vi "Newmark-GotoAll.vi"(0 "Table VRN IN":refnum<visa-resource-name>="COM9", 1 "BrasPesto":bool, 2 "Bool Refnum":refnum<vi>, 3 "LimXPesto":dbl, 7 "Notify?":bool, 11 "Error IN":errorcluster, 12 "Position X":dbl, 13 "Position Y":dbl, 14 "Position Z":dbl) -> (4 "Table VRN OUT":refnum<visa-resource-name>="COM9", 15 "Error OUT":errorcluster)   [LabVIEW 2019]
uses:
  Comm/SerialCommError.vi
panel:
  out "LimXPesto 2":dbl=54.5268 caption="Limit X avec Pesto" format="%.2f"
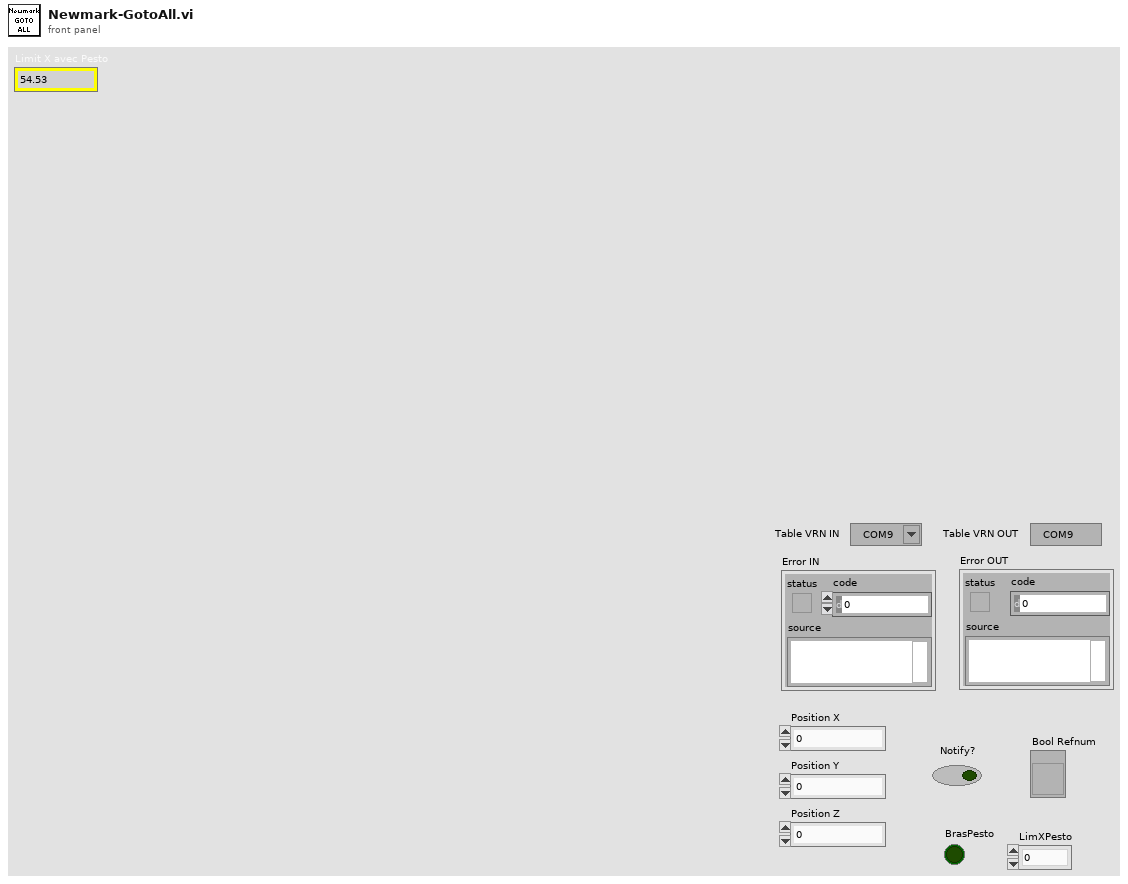
[diagram p1: front panel]
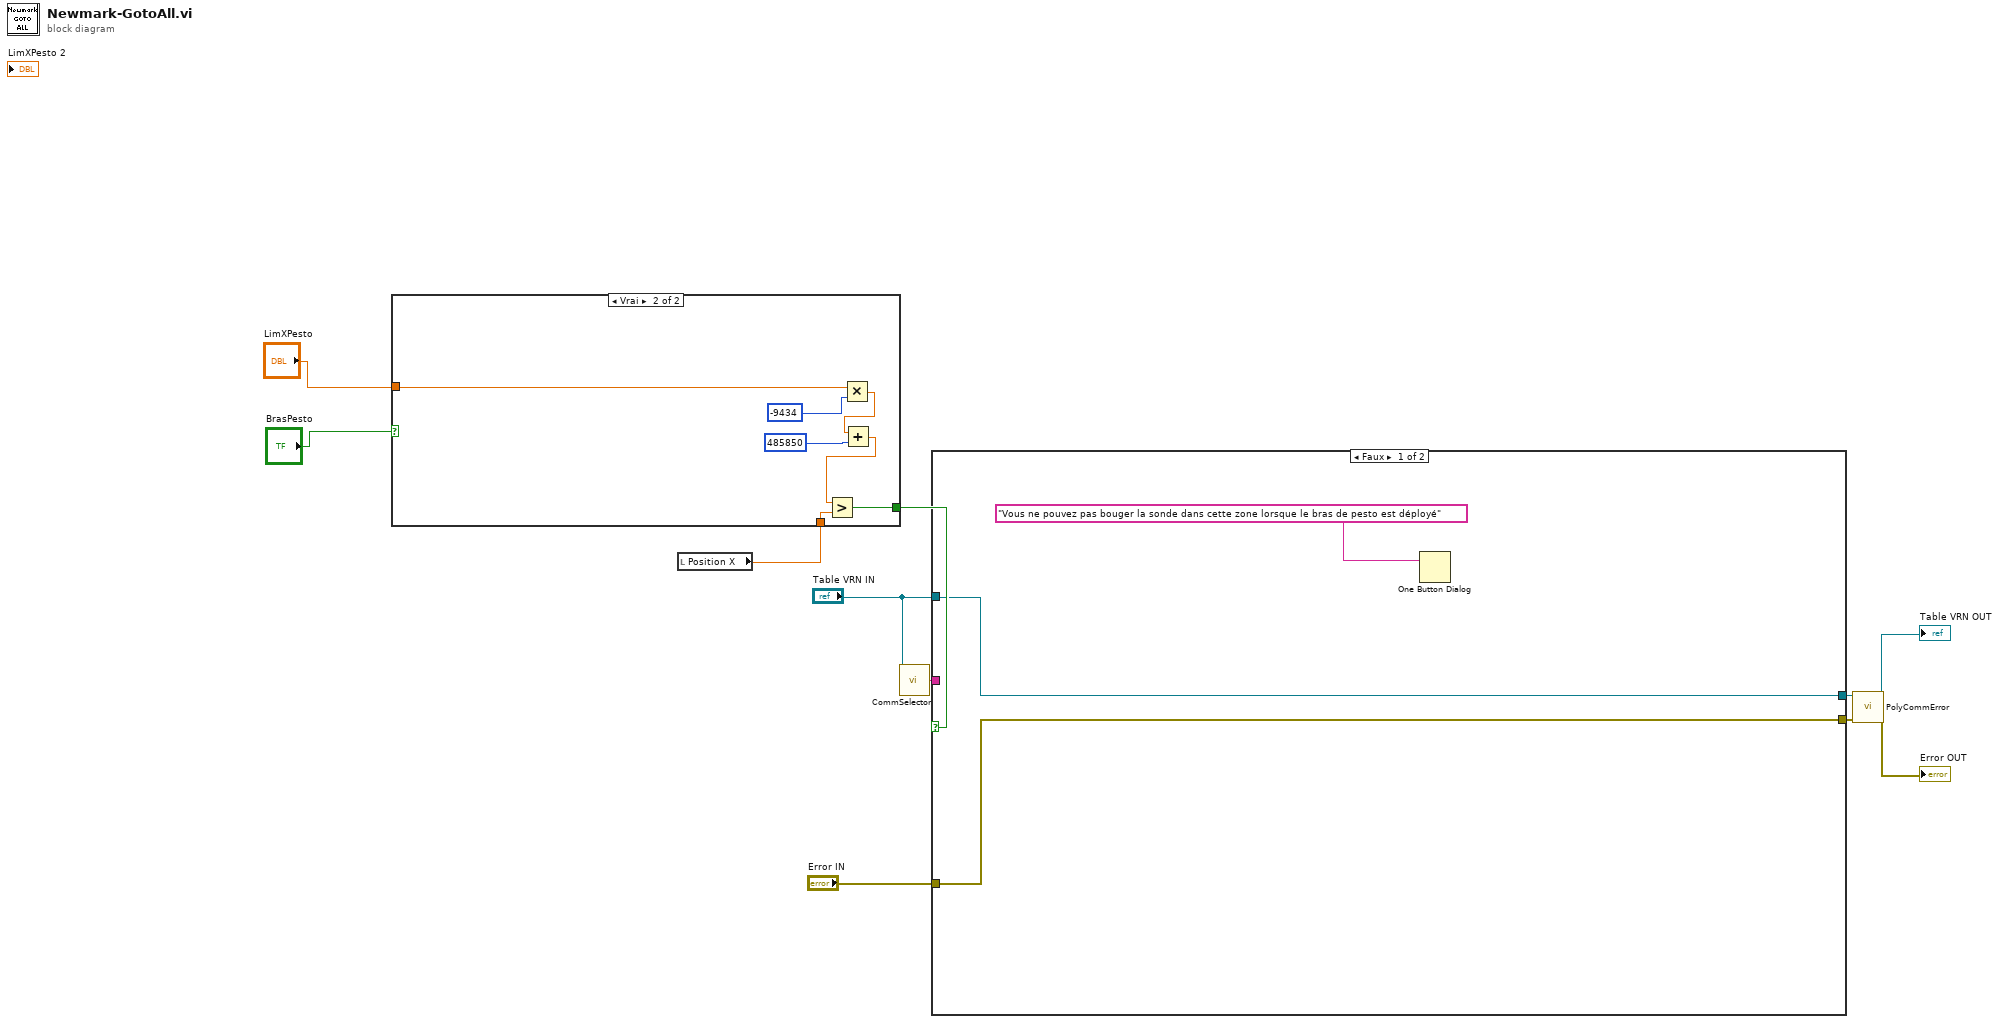
[diagram p0: block diagram]
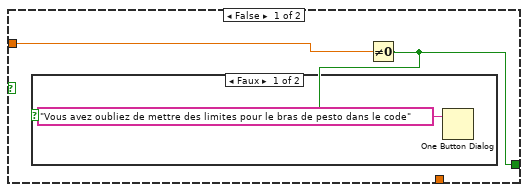
[diagram p2: hidden frame]
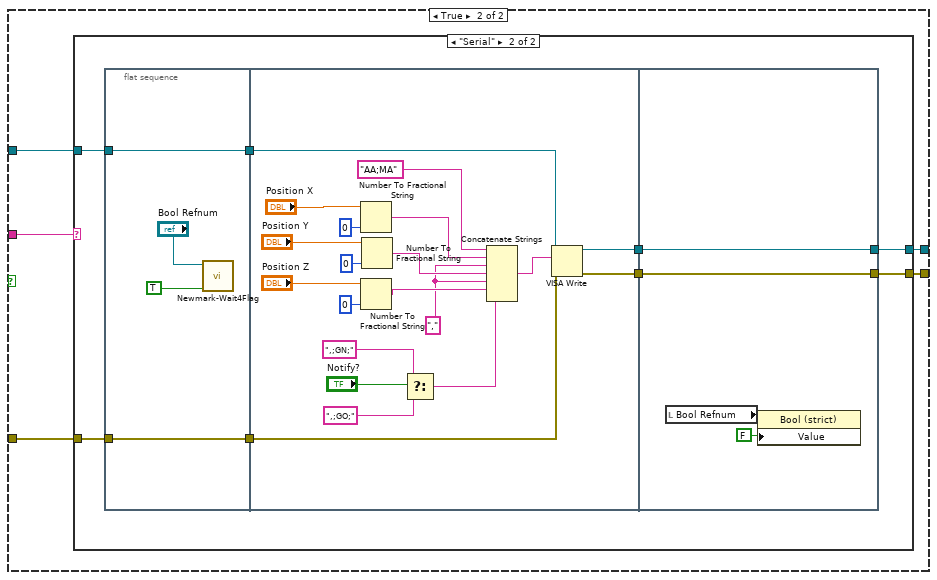
[diagram p4: hidden frame]
diagram:
  n1 = local read "Position X"() -> (w4:dbl)
  n2 = case shown="Vrai" "BrasPesto" {
    tunnel: w4 -> [_ w17]
    tunnel: [w12 w16] -> w3
    tunnel: "LimXPesto" -> [w13 w15]
    frame False {
      n3 = Not Equal To 0?(x=w13) -> (x != 0?=w12:bool)
      n4 = case shown="Faux" w12 {
        frame False {
          n5 = One Button Dialog(message="Vous avez oubliez de mettre des limites pour le bras de pesto dans le code") -> ()  [unwired: 1 in, 1 out]
        }
        frame True {
        }
      }
    }
    frame True {
      n6 = Multiply(x=w15, y=-9434) -> (x*y=w20:dbl)
      n7 = Add(x=w20, y=485850) -> (x+y=w18:dbl)
      n8 = Greater?(x=w18, y=w17) -> (0:w16:bool)
    }
  }
  n9 = call "CommSelector.vi"("VISA resource name"="Table VRN IN") -> ("CommType"=w5:string)  [unwired: 13 in, 1 out]
  n10 = case shown="Faux" w3 {
    tunnel: [w23 w29] -> w11
    tunnel: [w24 w28] -> w10
    tunnel: "Error IN" -> [w23 w27]
    tunnel: "Table VRN IN" -> [w24 w26]
    tunnel: w5 -> [_ w25]
    frame False {
      n11 = One Button Dialog(message="Vous ne pouvez pas bouger la sonde dans cette zone lorsque le bras de pesto est déployé") -> ()  [unwired: 1 in, 1 out]
    }
    frame True {
      n12 = case shown="\"Serial\"" w25 {
        tunnel: w26 -> [w31 w38]
        tunnel: w27 -> [w30 w36]
        tunnel: [w31 w35] -> w28
        tunnel: [w30 w33] -> w29
        frame "Unknown", Default {
        }
        frame "Serial" {
          n13 = flat-sequence {
            tunnel: [w41] -> w39
            tunnel: w38 -> [w41]
            tunnel: [w40] -> w37
            tunnel: w36 -> [w40]
            tunnel: w39 -> [w55]
            tunnel: w37 -> [w54]
            tunnel: [w53] -> w34
            tunnel: [w52] -> w32
            tunnel: [w65] -> w35
            tunnel: w34 -> [w65]
            tunnel: [w64] -> w33
            tunnel: w32 -> [w64]
            frame #0 {
              n14 = call "Newmark-Wait4Flag.vi"("Raise Flag ?"=TRUE, "Ctl Refnum IN"="Bool Refnum") -> ()  [unwired: 8 in, 2 out]
            }
            frame #1 {
              w44 = "," ("string")
              n15 = Number To Fractional String(number="Position X", precision (6)=i16 0) -> (F-format string=w60:string)  [unwired: 2 in]
              n16 = Number To Fractional String(number="Position Z", precision (6)=i16 0) -> (F-format string=w48:string)  [unwired: 2 in]
              n17 = Number To Fractional String(number="Position Y", precision (6)=i16 0) -> (F-format string=w49:string)  [unwired: 2 in]
              n18 = Select(t=",;GN;" ("string"), s="Notify?", f=",;GO;" ("string")) -> (s? t:f=w47:string)
              n19 = Concatenate Strings("AA;MA" ("string"), w60, w44, w49, w44, w48, w47) -> (w62:string)
              n20 = VISA Write(VISA resource name=w55, write buffer=w62, error in (no error)=w54) -> (VISA resource name out=w53:refnum<visa-resource-name>, error out=w52:errorcluster)  [unwired: 1 out]
            }
            frame #2 {
              n21 = local read "Bool Refnum"() -> (w67:refnum<vi>)
              n22 = property class="Bool (strict)"(reference=w67, "Value"=FALSE) -> ()  [unwired: 1 in, 2 out]
            }
          }
        }
      }
    }
  }
  n23 = call-poly "PolyCommError.vi"("VISA IN"=w10, "error IN"=w11) -> ("VISA OUT"=→"Table VRN OUT":refnum<visa-resource-name>, "error OUT"=→"Error OUT":errorcluster)  [unwired: 11 in, 1 out]
